vi "Read Gantry Head Vacuum.vi"(8 "error in":errorcluster, 10 "Inner/Outer":enum16{"Outer", "Inner"}(ring), 11 "Gantry in":refnum<class "Gantry Class.lvclass">) -> (0 "error out":errorcluster, 2 "On/Off":bool, 3 "Gantry out":refnum<class "Gantry Class.lvclass">)   [LabVIEW 2011, in "Gantry Class.lvclass"]
uses:
  Gantry Class.lvclass
  WorkTable Class/WorkTable Class.lvclass
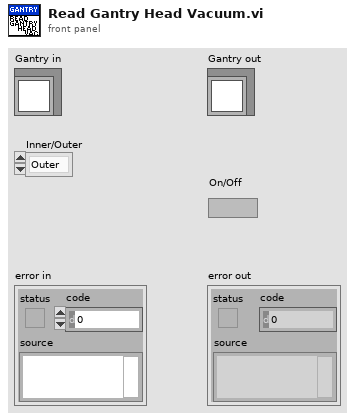
[diagram p1: front panel]
types:
  T1 = typedef "Worktable_Gantry Head.ctl" = cluster{"Current Tool":enum16{"None", "Grabber", "Picker", "Tool Setter"}, "Vacuum Channel Inner":i32, "Vacuum Channel Outer":i32}
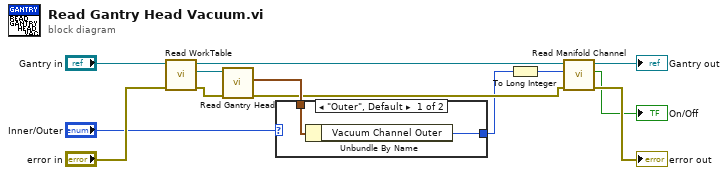
[diagram p0: block diagram]
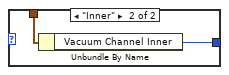
[diagram p2: hidden frame]
diagram:
  n1 = call-dynamic "Read WorkTable.vi"("error in"="error in", "Gantry Class in"="Gantry in") -> ("error out"=w4:errorcluster, "WorkTable Class.lvclass"=w7:refnum<class "WorkTable Class.lvclass">, "Gantry Class out"=w5:refnum<class "Gantry Class.lvclass">)  [unwired: 7 in]
  n2 = call-dynamic "Read Gantry Head.vi"("error in (no error)"=w4, "WorkTable Class in"=w7) -> ("error out"=w3:errorcluster, "Gantry Head"=w6:T1)  [unwired: 7 in, 1 out]
  n3 = case shown="\"Outer\", Default" "Inner/Outer" {
    tunnel: w6 -> [w15 w17]
    tunnel: [w14 w16] -> w2
    frame "Outer", Default {
      n4 = Unbundle By Name(w15) -> ("Vacuum Channel Outer"=w14:i32)
    }
    frame "Inner" {
      n5 = Unbundle By Name(w17) -> ("Vacuum Channel Inner"=w16:i32)
    }
  }
  n6 = To Long Integer(number=w2) -> (32bit integer=w1:i32)
  n7 = call-dynamic "Read Manifold Channel.vi"("error in"=w3, "Manifold Channel"=w1, "Gantry in"=w5) -> ("error out"=→"error out":errorcluster, "On/Off"=→"On/Off":bool, "Gantry out"=→"Gantry out":refnum<class "Gantry Class.lvclass">)  [unwired: 6 in]
